vi "Populate Available Wfms.vi"(4 "Full Path info":bool, 6 "Refresh List":bool, 8 "Error In":errorcluster, 9 "ListBox Variant":variant, 10 "CD Settings":T1={"CD Task Dependency"=18446744073709551615, "CD Task Dependency Ref"=18446744073709551615, "CD Task Available Wfms"=[], "CD Task Selected Wfms"=[], "Buffer Length (samples)"=0, "Min Enabled"=FALSE, "Max Enabled "=FALSE, "SP Enabled"=FALSE, "RMS Enabled"=FALSE, "Buffer Length (s)"=0.0, "Task Rate"=0.0, "Number of DAQ Chanels"=0} {"CD Task Dependency Ref" format="%.0x"; "CD Task Dependency" format="%.0x"}, 11 "CustomDevice Ref":T2 format="%.0x") -> (0 "Error Out":errorcluster, 1 "ListBox Variant":variant, 2 "CD Settings out":T1={"CD Task Dependency"=18446744073709551615, "CD Task Dependency Ref"=18446744073709551615, "CD Task Available Wfms"=[], "CD Task Selected Wfms"=[], "Buffer Length (samples)"=0, "Min Enabled"=FALSE, "Max Enabled "=FALSE, "SP Enabled"=FALSE, "RMS Enabled"=FALSE, "Buffer Length (s)"=0.0, "Task Rate"=0.0, "Number of DAQ Chanels"=0} {"CD Task Dependency Ref" format="%.0x"; "CD Task Dependency" format="%.0x"}, 3 "CustomDevice Ref":T2 format="%.0x", 5 "Number of DAQ Channels":u32 caption="# Ch's")   [LabVIEW 2017, in "Waveform-Processing-Custom-Device System Explorer.lvlib"]
doc: "This scans the selected waveform task and populates the discovered channel names into the \"Available Waveforms\" list. \n\nThis also populates the number of channels value"
uses:
  Waveform-Processing-Custom-Device System Explorer.lvlib
  <vilib>/NI Veristand/Custom Device API/Custom Device Item Ref.ctl
  Shared/Custom Device Settings.ctl
  NationalInstruments.VeriStand.SystemStorage
  NationalInstruments.VeriStand
  <userlib>/_OpenG.lib/array/array.llb/Remove Duplicates from 1D Array (String)__ogtk.vi
  <vilib>/NI VeriStand/Custom Device Tools/Custom Device Utility Library/Custom Device Utility Library.lvlib
  <vilib>/NI Veristand/Custom Device API/Custom Device API.lvlib
  Shared/Waveform-Processing-Custom-Device Shared.lvlib
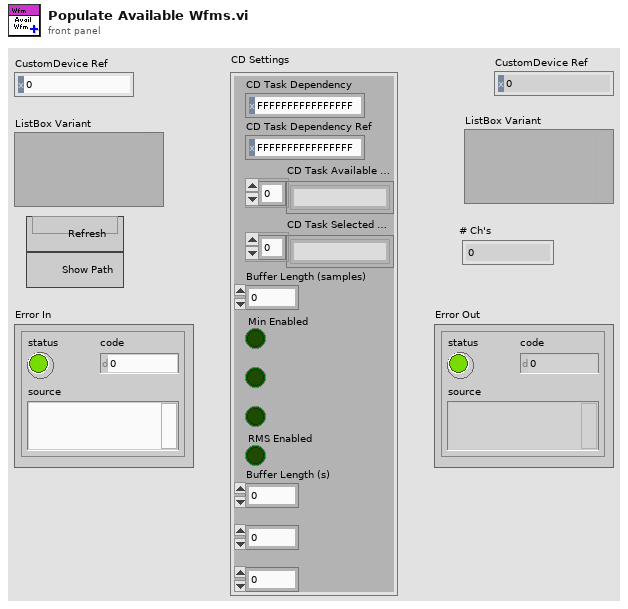
[diagram p1: front panel]
types:
  T1 = typedef "Waveform-Processing-Custom-Device Shared.lvlib/Custom Device Settings.ctl" = cluster{"CD Task Dependency":T2, "CD Task Dependency Ref":T2, "CD Task Available Wfms":string[], "CD Task Selected Wfms":string[], "Buffer Length (samples)":u32, "Min Enabled":bool, "Max Enabled ":bool, "SP Enabled":bool, "RMS Enabled":bool, "Buffer Length (s)":dbl, "Task Rate":dbl, "Number of DAQ Chanels":u32}
  T2 = typedef "Custom Device API.lvlib/Custom Device Item Ref.ctl" = u64
  T3 = typedef "Custom Device API.lvlib/Custom Device Pointer.ctl" = refnum<k24>
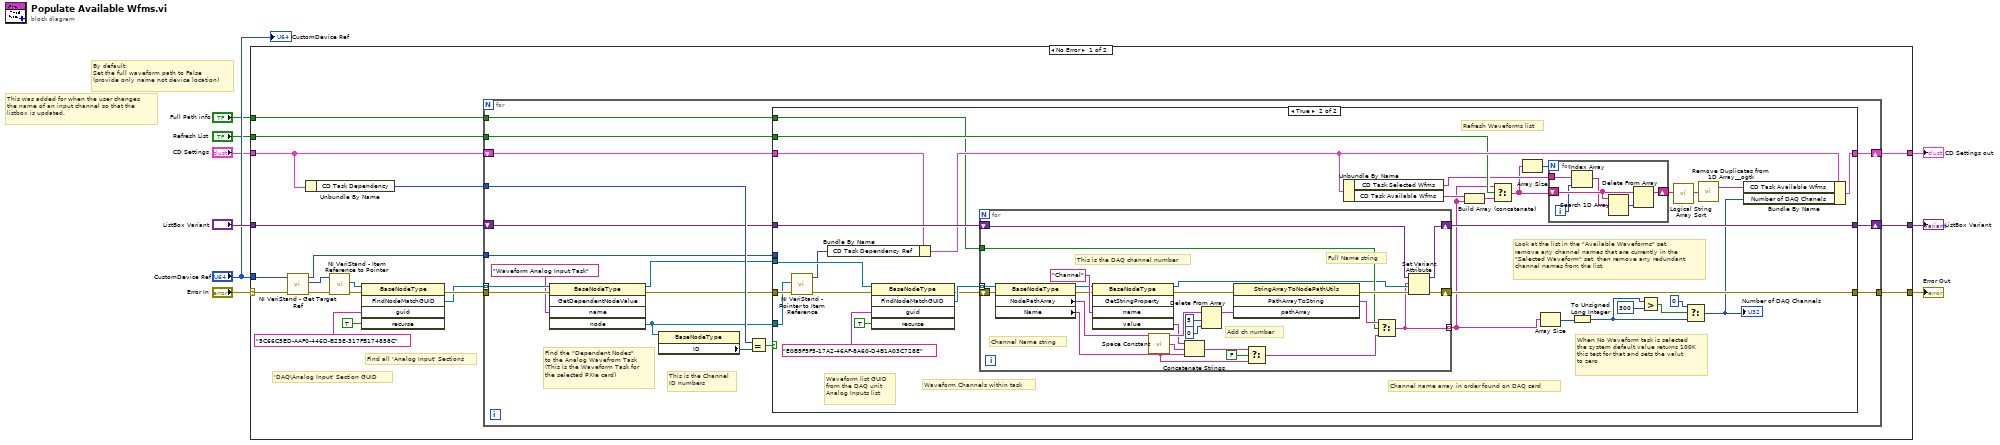
[diagram p0: block diagram]
diagram:
  # "This was added for when the user changes \nthe name of an input channel so that the \nlistbox is updated."
  # "By default:\nSet the full waveform path to False \n(provide only name not device location)"
  n1 = case shown="No Error" "Error In" {
    selector: "Error In" -> [w28 w113]
    tunnel: [w20 w113] -> w4
    tunnel: "CustomDevice Ref" -> [w17 _]
    tunnel: [w19 w112] -> w8
    tunnel: "ListBox Variant" -> [w18 w112]
    tunnel: "CD Settings" -> [w14 w111]
    tunnel: [w13 w111] -> w5
    tunnel: "Refresh List" -> [w11 _]
    tunnel: "Full Path info" -> [w10 _]
    frame No Error {
      # "'DAQ\\Analog Input' Section GUID"
      # "Find all 'Analog Input' Sections"
      n2 = call <vilib>:"NI VeriStand - Get Target Ref.vi"("error in"=w28, "Item Ref in"=w17) -> ("error out"=w27:errorcluster, "Target Ref"=w26:T2, "Item Ref out"=w16:T2)  [unwired: 6 in, 1 out]
      n3 = Unbundle By Name(w14) -> ("CD Task Dependency"=w15:T2)
      n4 = call <vilib>:"NI VeriStand - Item Reference to Pointer.vi"("error in (no error)"=w27, "Item Ref in"=w26) -> ("error out"=w24:errorcluster, "Node Pointer"=w25:T3)  [unwired: 6 in, 2 out]
      n5 = invoke class="BaseNodeType" method="FindNodeMatchGUID"(reference=w25, error in=w24, "guid"="5C66C5ED-AAF0-446D-B23E-317FB174858C" ("Item GUID"), "recurse"=TRUE ("Find All? (T)")) -> (error out=w21:errorcluster, "FindNodeMatchGUID"=w12:refnum<k24>[])  [unwired: 1 in, 3 out]
      n6 = for {
        tunnel: w15 -> [w45]
        tunnel: w12 -> [w44] mode=indexing
        tunnel: w21 -> [w43]
        tunnel: [w38] -> w20
        shift-right: [w37] -> w19
        shift-left: w18 -> [w36]
        tunnel: w16 -> [w35]
        shift-right: [w31] -> w13
        shift-left: w14 -> [w32]
        tunnel: w11 -> [w30]
        tunnel: w10 -> [w29]
        # "This is the Channel\nID numbers"
        # "Find the \"Dependent Nodes\" \nto the Analog Wavefrom Task\n(This is the Waveform Task for \nthe selected PXIe card)"
        n7 = invoke class="BaseNodeType" method="GetDependentNodeValue"(reference=w44, error in=w43, "name"="Waveform Analog Input Task" ("Property Name")) -> (reference out=w33:refnum<k24>, error out=w40:errorcluster, "node"=w34:refnum<k24>)  [unwired: 2 in, 2 out]
        n8 = property class="BaseNodeType"(reference=w34) -> ("ID"=w41:u64)  [unwired: 1 in, 2 out]
        n9 = Equal?(x=w45, y=w41) -> (x = y?=w39:bool)
        n10 = case shown="True" w39 {
          tunnel: w34 -> [_ w72]
          tunnel: w40 -> [w48 w73]
          tunnel: [w48 w76] -> w38
          tunnel: [w47 w75] -> w37
          tunnel: w36 -> [w47 w74]
          tunnel: w35 -> [_ _]
          tunnel: w33 -> [_ w71]
          tunnel: w32 -> [w46 w70]
          tunnel: [w46 w65] -> w31
          tunnel: w30 -> [_ w63]
          tunnel: w29 -> [_ w62]
          frame False {
          }
          frame True {
            # "When No Waveform task is selected\nthe system default value returns 100K\nthis test for that and sets the valut \nto zero"
            # "Channel name array in order found on DAQ card"
            # "Refresh Waveforms list"
            # "Look at the list in the \"Available Waveforms\" set, \nremove any channel names that are currently in the \n\"Selected Waveform\" set, then remove any redundant \nchannel names from the list."
            # "Waveform list GUID\nfrom the DAQ unit\nAnalog Inputs list"
            # "Waveform Channels within task"
            n11 = call <vilib>:"NI VeriStand - Pointer to Item Reference.vi"("error in (no error)"=w73, "Node Pointer"=w72) -> ("error out"=w68:errorcluster, "Item Ref out"=w69:T2)  [unwired: 8 in]
            n12 = Bundle By Name(cluster=w70, "CD Task Dependency Ref"=w69) -> (w66:T1)
            n13 = invoke class="BaseNodeType" method="FindNodeMatchGUID"(reference=w71, error in=w68, "guid"="E0B9F5F5-17A2-46AF-8A60-D4B1A03C728E", "recurse"=TRUE ("Find All? (T)")) -> (error out=w77:errorcluster, "FindNodeMatchGUID"=w78:refnum<k24>[])  [unwired: 1 in, 3 out]
            n14 = for {
              tunnel: w78 -> [w101] mode=indexing
              shift-right: [w98] -> w75
              shift-left: w74 -> [w97]
              shift-right: [w99] -> w76
              shift-left: w77 -> [w100]
              tunnel: [w81] -> w50 mode=indexing
              tunnel: w62 -> [w93]
              # "Add ch number"
              # "This is the DAQ channel number"
              # "Channel Name string"
              # "Full Name string"
              n15 = property class="BaseNodeType"(reference=w101, error in=w100) -> (reference out=w82:refnum<k24>, error out=w91:errorcluster, "NodePathArray"=w102:string[], "Name"=w83:string)
              n16 = invoke class="BaseNodeType" method="GetStringProperty"(reference=w82, error in=w91, "name"="Channel") -> (reference out=w89:refnum<k24>, error out=w90:errorcluster, "value"=w87:string)  [unwired: 2 in, 2 out]
              n17 = call <vilib>:"Space Constant.vi"() -> ("String"=w88:string)
              n18 = Concatenate Strings(w87, w88, w83) -> (w85:string)
              n19 = Delete From Array(array=w102, length=5, index=0) -> (array with subset deleted=w95:string[])  [unwired: 1 out]
              n20 = invoke class="StringArrayToNodePathUtils" method="PathArrayToString"(error in=w90, "pathArray"=w95) -> (error out=w96:errorcluster, "PathArrayToString"=w94:string)  [unwired: 2 in, 2 out]
              n21 = Select(t=w85, s=FALSE, f=w83) -> (s? t:f=w84:string)
              n22 = Select(t=w94, s=w93, f=w84) -> (s? t:f=w81:string)
              n23 = Set Variant Attribute(Variant=w97, name=w81, value=w89, error in=w96) -> (Variant out=w98:variant, error out=w99:errorcluster)  [unwired: 1 out]
            }
            n24 = Unbundle By Name(w66) -> ("CD Task Selected Wfms"=w61:string[], "CD Task Available Wfms"=w67:string[])
            n25 = Build Array (concatenate)(w67, w50) -> (w64:string[])
            n26 = Select(t=w50, s=w63, f=w64) -> (s? t:f=w60:string[])
            n27 = Array Size(array=w60) -> (size(s)=w59:i32)
            n28 = Array Size(array=w50) -> (size(s)=w52:i32)
            n29 = for {
              N: w59 -> [_]
              tunnel: w61 -> [w109]
              shift-right: [w107] -> w57
              shift-left: w60 -> [w110]
              i -> [w105]
              n30 = Index Array(array=w109, index=w105) -> (element=w106:string)
              n31 = Search 1D Array(1D array=w110, element=w106) -> (index of element=w108:i32)  [unwired: 1 in]
              n32 = Delete From Array(array=w110, index=w108) -> (array with subset deleted=w107:string[])  [unwired: 1 in, 1 out]
            }
            n33 = To Unsigned Long Integer(number=w52) -> (unsigned 32bit integer=w49:u32)
            n34 = Greater?(x=w49, y=u32 300) -> (0:w54:bool)
            n35 = call "Logical String Array Sort.vi"("Unsorted List"=w57) -> ("Sorted List"=w58:string[])  [unwired: 18 in]
            n36 = Select(t=u32 0, s=w54, f=w49) -> (s? t:f=w51:u32)
            "Number of DAQ Channels" <- w51
            n37 = call-poly <userlib>:"Remove Duplicates from 1D Array__ogtk.vi"("Input Array"=w58) -> ("Output Array"=w56:string[])  [unwired: 1 out]
            n38 = Bundle By Name(cluster=w66, "CD Task Available Wfms"=w56, "Number of DAQ Chanels"=w51) -> (w65:T1)
          }
        }
      }
    }
    frame Error {
    }
  }
  "ListBox Variant" <- w8
  "CD Settings out" <- w5
  "Error Out" <- w4
  "CustomDevice Ref" <- "CustomDevice Ref"
